vi "Triggered Acquisition.vi"(0 "RedPitaya TCP connection in":refnum<k5>, 2 "Trigger Mode":string(combo), 5 "error in":errorcluster, 12 "timeout ms (2000)":i32=2000) -> (14 "RedPitaya TCP connection out":refnum<k5>, 19 "error out":errorcluster)   [LabVIEW 2010, in "RedPitaya.lvlib"]
doc: "Enables triggered data acquisition and sets the trigger mode."
uses:
  RedPitaya.lvlib
panel:
  in  "milliseconds to wait":u32
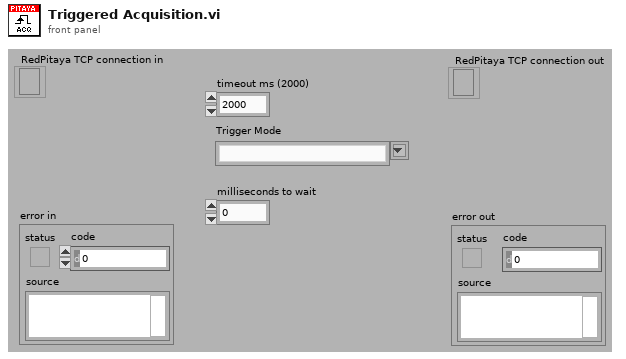
[diagram p1: front panel]
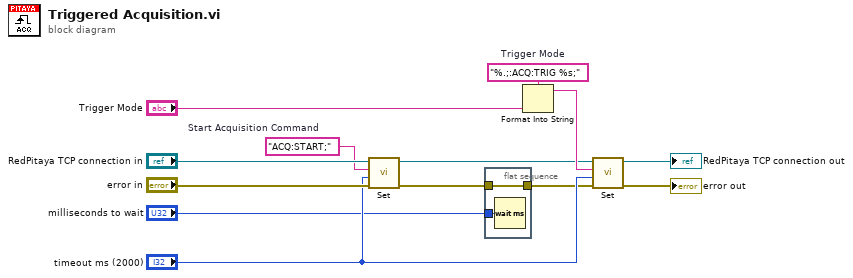
[diagram p0: block diagram]
diagram:
  w5 = "ACQ:START;"  # Start Acquisition Command
  w12 = "%.;:ACQ:TRIG %s;"  # Trigger Mode
  n1 = call "Set.vi"("error in"="error in", "timeout ms (2000)"="timeout ms (2000)", "SCPI Message"=w5, "RedPitaya connection in"="RedPitaya TCP connection in") -> ("error out"=w2:errorcluster, "RedPitaya connection out"=w6:refnum<k5>)  [unwired: 5 in, 1 out]
  n2 = flat-sequence {
    tunnel: "milliseconds to wait" -> [w15]
    tunnel: w2 -> [w14]
    tunnel: [w14] -> w1
    frame #0 {
      n3 = Wait (ms)(milliseconds to wait=w15) -> ()  [unwired: 1 out]
    }
  }
  n4 = Format Into String(format string=w12, "Trigger Mode") -> (resulting string=w13:string)  [unwired: 2 in, 1 out]
  n5 = call "Set.vi"("error in"=w1, "timeout ms (2000)"="timeout ms (2000)", "SCPI Message"=w13, "RedPitaya connection in"=w6) -> ("error out"=→"error out":errorcluster, "RedPitaya connection out"=→"RedPitaya TCP connection out":refnum<k5>)  [unwired: 5 in, 1 out]
